vi "Limit.vi"(0 "VisaCluster":T1, 7 "Limit":bool, 11 "error in (no error)":errorcluster) -> (4 "VisaCluster":T1, 8 "Answer":string, 10 "Limit":bool, 15 "error out":errorcluster)   [LabVIEW 2014, in "FH 55.lvlib"]
doc: "This VI sets the Limit ON or OFF.\n\nDiese VI Limit wird verwendet, um die Limit-Funktion ein- und auszuschalten. Die Limit-Funktion gibt ein optisches Signal, wenn der Messwert außerhalb oder innerhalb eines definierten Bereiches liegt."
uses:
  FH 55.lvlib
  TypeDef/VisaCluster.ctl
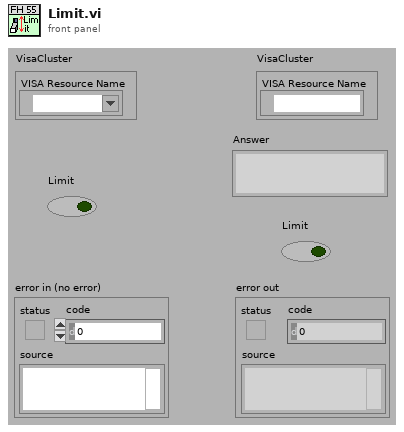
[diagram p1: front panel]
types:
  T1 = typedef "FH 55.lvlib/VisaCluster.ctl" = cluster{"VISA Resource Name":refnum<visa-resource-name>}
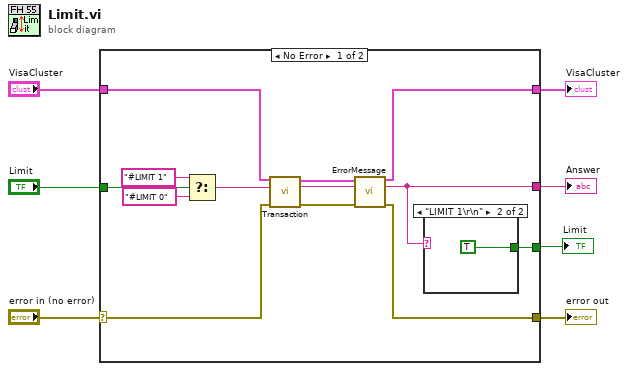
[diagram p0: block diagram]
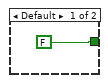
[diagram p2: hidden frame]
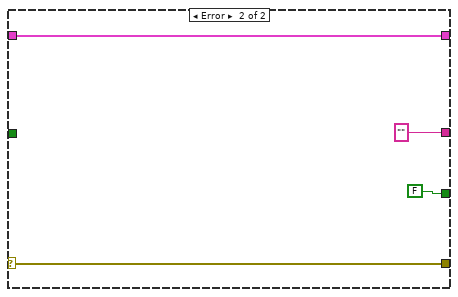
[diagram p3: hidden frame]
diagram:
  n1 = case shown="No Error" "error in (no error)" {
    selector: "error in (no error)" -> [w13 w25]
    tunnel: "VisaCluster" -> [w15 w26]
    tunnel: "Limit" -> [w20 _]
    tunnel: [w17 w26] -> w3
    tunnel: [w16 w25] -> w5
    tunnel: [w10 ""] -> w4
    tunnel: [w8 FALSE] -> w1
    frame No Error {
      n2 = Select(t="#LIMIT 1", s=w20, f="#LIMIT 0") -> (s? t:f=w14:string)
      n3 = call "Transaction.vi"("VisaCluster"=w15, "Command"=w14, "error in (no error)"=w13) -> ("VisaCluster"=w11:T1, "Answer"=w9:string, "error out"=w12:errorcluster)  [unwired: 9 in, 1 out]
      n4 = call "ErrorMessage.vi"("VisaCluster"=w11, "Message In"=w9, "error in (no error)"=w12) -> ("VisaCluster"=w17:T1, "Message Out"=w10:string, "error out"=w16:errorcluster)  [unwired: 10 in]
      n5 = case shown="\"LIMIT 1\\r\\n\"" w10 {
        tunnel: [FALSE TRUE] -> w8
        frame Default {
        }
        frame "LIMIT 1\r\n" {
        }
      }
    }
    frame Error {
    }
  }
  "error out" <- w5
  "Answer" <- w4
  "VisaCluster" <- w3
  "Limit" <- w1
